vi "Get Image.vi"(8 "error in (no error)":errorcluster, 11 "Image Acquisition in":refnum<class "Simulation.lvclass">) -> (0 "error out":errorcluster, 2 "Image Reference":T1, 3 "Image Acquisition out":refnum<class "Simulation.lvclass">)   [LabVIEW 2018, in "Simulation.lvclass"]
uses:
  Simulation.lvclass
  <vilib>/vision/Image Controls.llb/IMAQ Image.ctl
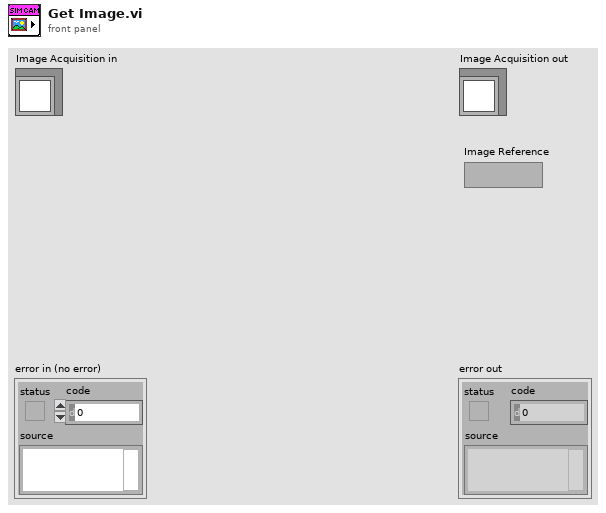
[diagram p1: front panel]
types:
  T1 = typedef "IMAQ Image.ctl" = refnum<image>
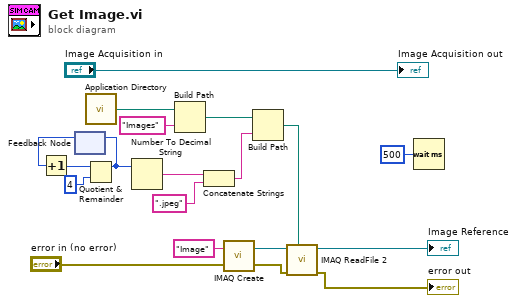
[diagram p0: block diagram]
diagram:
  n1 = feedback #1() -> (w5:i32)  [unwired: 1 in]
  n2 = Increment(x=w5) -> (x+1=w4:i32)
  n3 = call <vilib>:"Application Directory.vi"() -> ("Application Directory"=w15:path)
  n4 = Quotient & Remainder(x=w4, y=4) -> (x-y*floor(x/y)=w1:i32)  [unwired: 1 out]
  n5 = feedback-in #1(w1) -> ()
  n6 = Number To Decimal String(number=w1) -> (decimal integer string=w9:string)  [unwired: 1 in]
  n7 = Build Path(base path=w15, name or relative path="Images") -> (appended path=w7:path)
  n8 = Concatenate Strings(w9, ".jpeg" ("string")) -> (w6:string)
  n9 = call "IMAQ Create"("Image Name"="Image", "error in (no error)"="error in (no error)") -> ("New Image"=w17:T1, "error out"=w12:errorcluster)  [unwired: 3 in]
  n10 = Build Path(base path=w7, name or relative path=w6) -> (appended path=w3:path)
  n11 = call "IMAQ ReadFile 2"("File Path"=w3, "error in (no error)"=w12, "Image"=w17) -> ("error out"=→"error out":errorcluster, "Image Out"=→"Image Reference":T1)  [unwired: 4 in, 3 out]
  n12 = Wait (ms)(milliseconds to wait=u32 500) -> ()  [unwired: 1 out]
  "Image Acquisition out" <- "Image Acquisition in"
